vi "Terminal Relation Msg Output.vi"() -> (2 "Terminal Relation (Msg Output)":T1)   [LabVIEW 2020, in "_Rescript.lvlib" / "Msg.lvlib" / "Msg.lvclass"]
uses:
  Msg.lvclass
  Terminal Relation.ctl
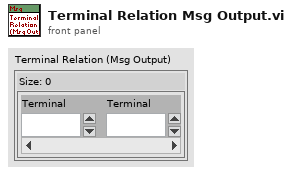
[diagram p1: front panel]
types:
  T1 = typedef "_Rescript.lvlib/Msg.lvlib/Msg.lvclass/Terminal Relation.ctl" = map{i32, i32}
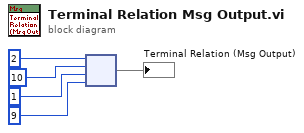
[diagram p0: block diagram]
diagram:
  n1 = node(2 ("Numeric"), 10 ("Numeric"), 1 ("Numeric"), 9 ("Numeric")) -> (→"Terminal Relation (Msg Output)":map{i32, i32})
